vi "Prepare Path.vi"(8 "error in (no error)":errorcluster, 9 "Extenssion":string, 10 "File Path in":path, 11 "Report Plugin In":refnum<class "Report Plugin.lvclass">) -> (0 "error out":errorcluster, 2 "Modified Path":path, 3 "Report Plugin Out":refnum<class "Report Plugin.lvclass">)   [LabVIEW 2020, in "Report Plugin.lvclass"]
doc: "If a relative path, convert to the full directory.\nIf directory, generate a file name with the given extenssion.\nIf file exists, generate next with incrementing index.\n\n<b>Developed by:</b>\nDaniel Coons, TSC"
uses:
  Report Plugin.lvclass
  C:/git/astemes-lunit/source/Framework/Report Plugin/Report Plugin.lvclass
  C:/git/astemes-lunit/source/Framework/Plugin/Plugin.lvclass
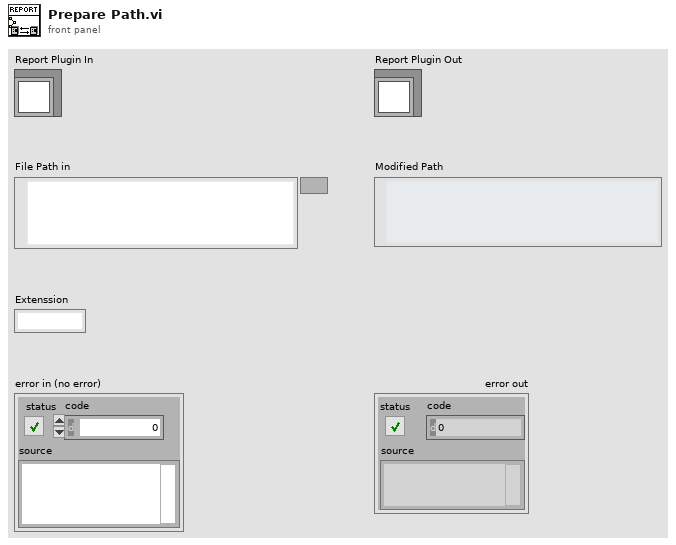
[diagram p1: front panel]
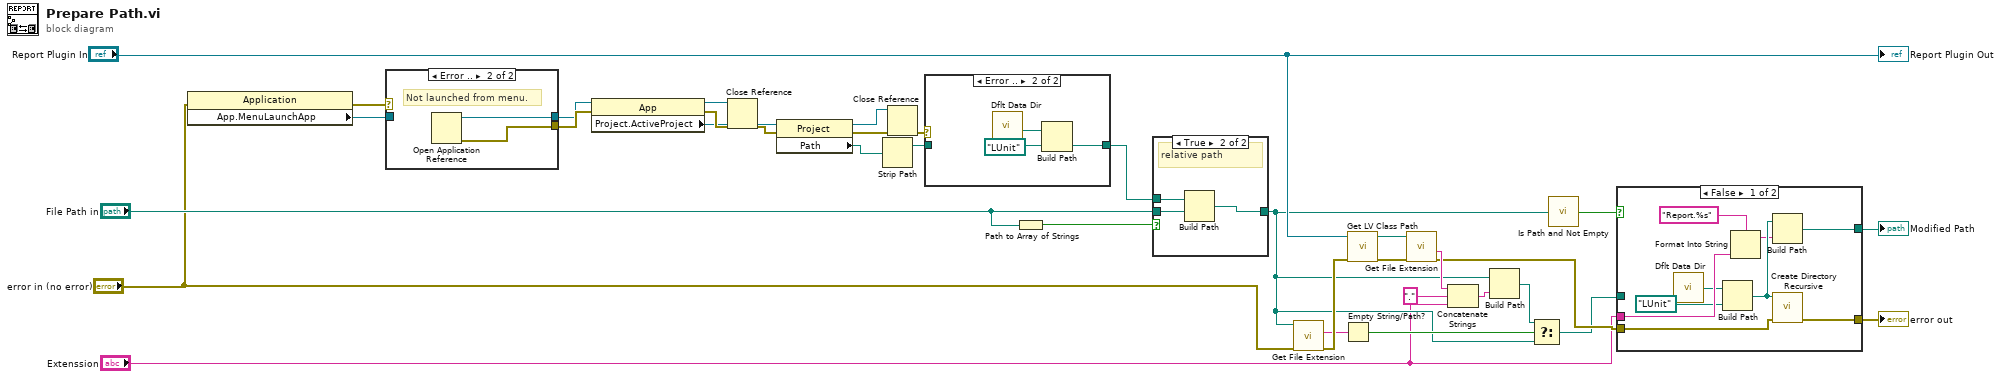
[diagram p0: block diagram]
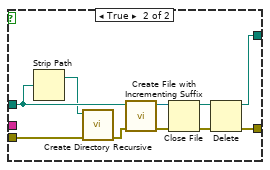
[diagram p5: hidden frame]
diagram:
  n1 = property class="Application"(error in="error in (no error)") -> (error out=w23:errorcluster, "App.MenuLaunchApp"=w24:refnum<vi>)  [unwired: 1 in, 1 out]
  n2 = case shown="Error .." w23 {
    selector: w23 -> [w35 _]
    tunnel: [w36 w38] -> w26
    tunnel: w24 -> [w36 _]
    tunnel: [w35 w37] -> w29
    frame No Error {
      # "Launch from menu"
    }
    frame Error {
      # "Not launched from menu."
      n3 = Open Application Reference() -> (0:w37:errorcluster, 3:w38:refnum<vi>)  [unwired: 4 in]
    }
  }
  n4 = property class="App"(reference=w26, error in=w29) -> (reference out=w28:refnum<vi>, error out=w30:errorcluster, "Project.ActiveProject"=w27:refnum<vi>)
  n5 = Close Reference(reference=w28, error in (no error)=w30) -> (error out=w25:errorcluster)
  n6 = property class="Project"(reference=w27, error in=w25) -> (reference out=w31:refnum<vi>, error out=w32:errorcluster, "Path"=w4:path)
  n7 = Strip Path(path=w4) -> (stripped path=w1:path)  [unwired: 1 out]
  n8 = Close Reference(reference=w31, error in (no error)=w32) -> (error out=w5:errorcluster)
  n9 = case shown="Error .." w5 {
    tunnel: w1 -> [w39 _]
    tunnel: [w39 w42] -> w3
    frame No Error {
    }
    frame Error {
      n10 = call <vilib>:"Dflt Data Dir.vi"() -> ("App:Default Data Directory"=w41:path)
      n11 = Build Path(base path=w41, name or relative path=path "LUnit") -> (appended path=w42:path)
    }
  }
  n12 = Path to Array of Strings(0:"File Path in") -> (1:w34:bool)  [unwired: 1 out]
  n13 = case shown="True" w34 {
    tunnel: "File Path in" -> [w43 w44]
    tunnel: [w43 w45] -> w7
    tunnel: w3 -> [_ w46]
    frame False {
      # "absolute path"
    }
    frame True {
      # "relative path"
      n14 = Build Path(base path=w46, name or relative path=w44) -> (appended path=w45:path)
    }
  }
  n15 = call <vilib>:"Get File Extension.vi"("error in (no error)"="error in (no error)", "file"=w7) -> ("error out"=w15:errorcluster, "lowercase file extension"=w14:string)  [unwired: 5 in, 3 out]
  n16 = Empty String/Path?(string/path=w14) -> (empty?=w13:bool)
  n17 = call <vilib>:"Get LV Class Path.vi"("error in (no error)"=w15, "object"="Report Plugin In") -> ("error out"=w22:errorcluster, "class path"=w21:path)  [unwired: 8 in]
  n18 = call <vilib>:"Get File Extension.vi"("error in (no error)"=w22, "file"=w21) -> ("error out"=w11:errorcluster, "filename without extension"=w20:string)  [unwired: 5 in, 3 out]
  n19 = Concatenate Strings(w20, "." ("string"), "Extenssion") -> (w18:string)
  n20 = Build Path(base path=w7, name or relative path=w18) -> (appended path=w17:path)
  n21 = Select(t=w17, s=w13, f=w7) -> (s? t:f=w10:path)
  n22 = call <vilib>:"Is Path and Not Empty.vi"("path"=w7) -> ("Is Path and Not Empty?"=w12:bool)  [unwired: 4 in]
  n23 = case shown="False" w12 {
    tunnel: w10 -> [_ w62]
    tunnel: [w55 w58] -> w9
    tunnel: w11 -> [w54 w59]
    tunnel: [w53 w56] -> w8
    tunnel: "Extenssion" -> [w51 _]
    frame False {
      n24 = call <vilib>:"Dflt Data Dir.vi"() -> ("App:Default Data Directory"=w47:path)
      n25 = Build Path(base path=w47, name or relative path=path "LUnit") -> (appended path=w52:path)
      n26 = Format Into String(format string="Report.%s", w51) -> (resulting string=w50:string)  [unwired: 2 in, 1 out]
      n27 = Build Path(base path=w52, name or relative path=w50) -> (appended path=w53:path)
      n28 = call <vilib>:"Create Directory Recursive.vi"("error in (no error)"=w54, "directory"=w52) -> ("error out"=w55:errorcluster)  [unwired: 3 in, 2 out]
    }
    frame True {
      n29 = Strip Path(path=w62) -> (stripped path=w61:path)  [unwired: 1 out]
      n30 = call <vilib>:"Create Directory Recursive.vi"("error in (no error)"=w59, "directory"=w61) -> ("error out"=w60:errorcluster)  [unwired: 3 in, 2 out]
      n31 = call <vilib>:"Create File with Incrementing Suffix.vi"("error in (no error)"=w60, "file path"=w62) -> ("error out"=w63:errorcluster, "refnum out"=w64:refnum<file>)  [unwired: 7 in, 1 out]
      n32 = Close File(refnum=w64, error in=w63) -> (path=w57:path, error out=w65:errorcluster)
      n33 = Delete(path (use dialog)=w57, error in=w65) -> (deleted path=w56:path, error out=w58:errorcluster)  [unwired: 3 in, 1 out]
    }
  }
  "Modified Path" <- w8
  "error out" <- w9
  "Report Plugin Out" <- "Report Plugin In"
